vi "Conversions.vi"() -> ()   [LabVIEW 2020]
panel:
  in  "u16 2":u16
  out "u8 2":u8
  out "u16":u16
  in  "u8":u8
  # "N"
  # "Rolled Off"
  # "255+N"
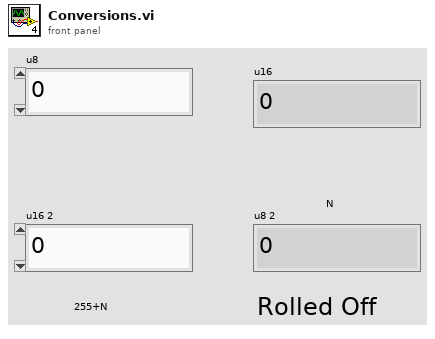
[diagram p1: front panel]
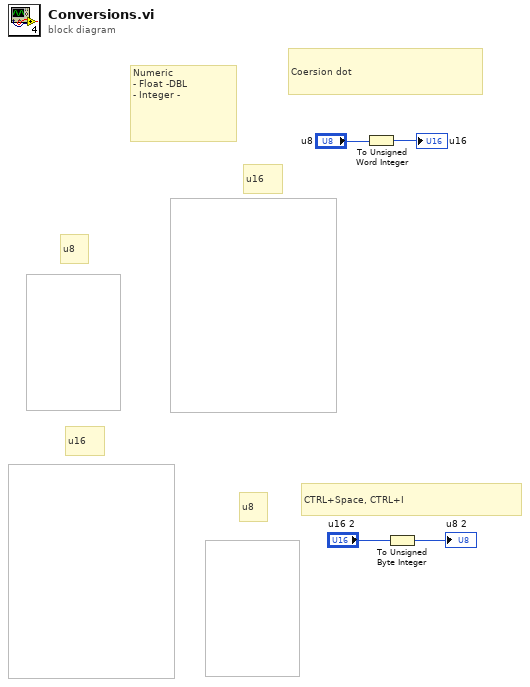
[diagram p0: block diagram]
diagram:
  # "CTRL+Space, CTRL+I"
  # "Coersion dot"
  # "u8"
  # "u16"
  # "u16"
  # "u8"
  # "Numeric\n- Float -DBL\n- Integer -"
  n1 = To Unsigned Word Integer(number="u8") -> (unsigned 16bit integer=→"u16":u16)
  n2 = To Unsigned Byte Integer(number="u16 2") -> (unsigned 8bit integer=→"u8 2":u8)
